vi "VI Tester Project API Create New TestSuite.vi"(8 "error in":errorcluster, 11 "Object":T1) -> (0 "error out":errorcluster)   [LabVIEW 2009]
uses:
  VITester Project Item Ref.ctl
  VI Tester Project API Method Selector - Enum.ctl
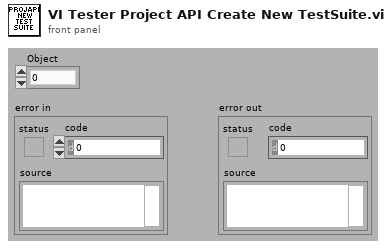
[diagram p1: front panel]
types:
  T1 = typedef "VITester Project Item Ref.ctl" = u64
  T2 = typedef "VI Tester Project API Method Selector - Enum.ctl" = enum16{"Open VI Tester", "Run All Tests", "Create New TestCase", "Create New TestSuite"}
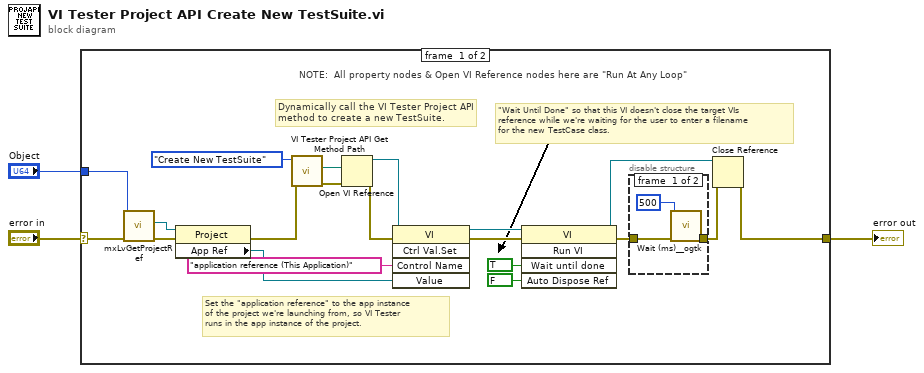
[diagram p0: block diagram]
diagram:
  n1 = case shown="No Error" "error in" {
    selector: "error in" -> [w10 w28]
    tunnel: [w23 w28] -> w3
    tunnel: "Object" -> [w20 _]
    frame #0 {
      # "\"Wait Until Done\" so that this VI doesn't close the target VIs\nreference while we're waiting for the user to enter a filename\nfor the new TestCase class."
      # "Set the \"application reference\" to the app instance\nof the project we're launching from, so VI Tester\nruns in the app instance of the project."
      # "Dynamically call the VI Tester Project API\nmethod to create a new TestSuite."
      # "NOTE:  All property nodes & Open VI Reference nodes here are \"Run At Any Loop\""
      n2 = call "mxLvGetProjectRef.vi"("error in"=w10, "Item"=w20) -> ("error out"=w11:errorcluster, "Project Refnum"=w12:refnum<vi>)  [unwired: 7 in, 1 out]
      n3 = property class="Project"(reference=w12, error in=w11) -> (error out=w5:errorcluster, "App Ref"=w6:refnum<vi>)  [unwired: 1 out]
      n4 = call "VI Tester Project API Get Method Path.vi"("error in (no error)"=w5, "Project API Method"=VI_Tester_Project_API_Method_Selector_-_Enum."Create New TestSuite") -> ("error out"=w8:errorcluster, "Path to VI Tester Project API Proxy VI"=w21:path)  [unwired: 8 in]
      n5 = Open VI Reference(vi path=w21, error in (no error)=w8) -> (vi reference=w4:refnum<vi>, error out=w16:errorcluster)  [unwired: 4 in]
      n6 = invoke class="VI" method="Ctrl Val.Set"(reference=w4, error in=w16, "Control Name"="application reference (This Application)", "Value"=w6) -> (reference out=w14:refnum<vi>, error out=w15:errorcluster)  [unwired: 1 in, 3 out]
      n7 = invoke class="VI" method="Run VI"(reference=w14, error in=w15, "Wait until done"=TRUE ("Wait Until Done"), "Auto Dispose Ref"=FALSE ("Auto Dispose Reference")) -> (reference out=w7:refnum<vi>, error out=w17:errorcluster)  [unwired: 1 in, 3 out]
      n8 = disable-structure shown="Enabled" {
        disable-tunnel: [w26 w27] -> w22
        disable-tunnel: w17 -> [w25 w27]
        frame #0 {
          n9 = call <userlib>:"Wait (ms)__ogtk.vi"("error in (no error)"=w25, "milliseconds to wait"=u32 500) -> ("error out"=w26:errorcluster)  [unwired: 8 in, 1 out]
        }
        frame #1 {
        }
      }
      n10 = Close Reference(reference=w7, error in (no error)=w22) -> (error out=w23:errorcluster)
    }
    frame #1 {
    }
  }
  "error out" <- w3
